vi "Measurement_Tab_Enabling.vi"(7 "Page_Label":u16(ring), 8 "Error in":errorcluster, 10 "Page_State":T1(ring)=enum."Page Disabled & Grayed", 11 "TabControl in":refnum<vi>) -> (0 "Error out":errorcluster)   [LabVIEW 2017]
doc: "Controls the Main Tab Control of the Benni_Prüfstand VI. Used for making sure that the Verfiy Channel Control button is pressed before measurement commences"
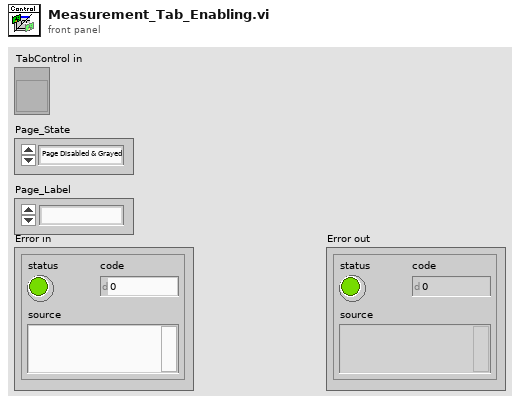
[diagram p1: front panel]
types:
  T1 = enum32{"Page Enabled", "Page Disabled", "Page Disabled & Grayed"}
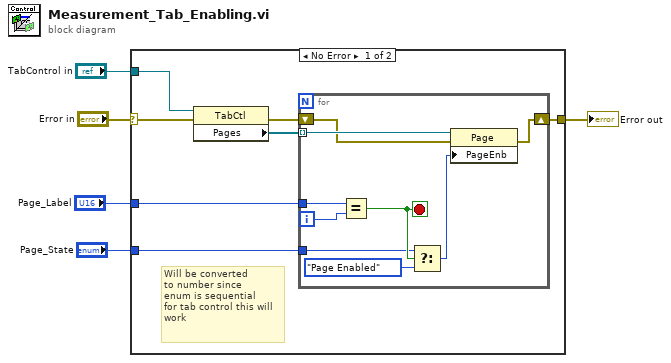
[diagram p0: block diagram]
diagram:
  n1 = case shown="No Error" "Error in" {
    selector: "Error in" -> [w10 w22]
    tunnel: "TabControl in" -> [w12 _]
    tunnel: [w8 w22] -> w3
    tunnel: "Page_Label" -> [w7 _]
    tunnel: "Page_State" -> [w6 _]
    frame No Error {
      # "Will be converted\nto number since\nenum is sequential\nfor tab control this will\nwork"
      n2 = property on="Property Node" class="TabCtl"(reference=w12, error in=w10) -> (error out=w9:errorcluster, "Pages"=w11:refnum<vi>[])  [unwired: 1 out]
      n3 = for {
        tunnel: w11 -> [w16] mode=indexing
        tunnel: w7 -> [w18]
        shift-right: [w19] -> w8
        shift-left: w9 -> [w14]
        tunnel: w6 -> [w13]
        i -> [w17]
        stop <- w15 stop-if-true
        n4 = Equal?(x=w18, y=w17) -> (x = y?=w15:bool)
        n5 = Select(t=w13, s=w15, f=T1."Page Enabled" ("Page Enabled State")) -> (s? t:f=w20:T1)
        n6 = property class="Page"(reference=w16, error in=w14, "PageEnb"=w20) -> (error out=w19:errorcluster)  [unwired: 1 out]
      }
    }
    frame Error {
    }
  }
  "Error out" <- w3
